vi "Benchmark DMA.vi"() -> ()   [LabVIEW 2016]
uses:
  Controls/Throughput Metrics.ctl
  Controls/Overhead Metrics.ctl
panel:
  in  "Driver":enum16{"Old Driver", "New Driver"}(ring)=enum."New Driver"
  in  "Tab Control":T1(tab)
  out "Channel Counts":i32[](array[numeric])=[1, 10, 100, 1000, 10000, 100000]
  out "Block Write":T2[](array[typedef]) {"Transfer Rate" format="%.2pB/s"; "Duration Std. Dev." format="%.0f µs"; "Duration Average" format="%.0f µs"}
  out "Block Read":T2[](array[typedef]) {"Transfer Rate" format="%.2pB/s"; "Duration Std. Dev." format="%.0f µs"; "Duration Average" format="%.0f µs"}
  out "Scatter-Gather Write":T2[](array[typedef]) {"Transfer Rate" format="%.2pB/s"; "Duration Std. Dev." format="%.0f µs"; "Duration Average" format="%.0f µs"}
  out "Scatter-Gather Read":T2[](array[typedef]) {"Transfer Rate" format="%.2pB/s"; "Duration Std. Dev." format="%.0f µs"; "Duration Average" format="%.0f µs"}
  in  "Tab Control Histograms":enum32{"Block Write", "Page 2"}(tab)
  out "Block Write 100000":T3(graph)
  out "Block Write 10000":T3(graph)
  out "Block Write 1000":T3(graph)
  out "Block Write 100":T3(graph)
  out "Block Write 10":T3(graph)
  out "Block Write 1":T3(graph)
  out "Write Overhead":T4 {"Duration Scatter-Gather" format="%.0f µs"; "Duration N Blocks" format="%.0f µs"; "Duration 1 Block" format="%.0f µs"}
  out "Read Overhead":T4 {"Duration Scatter-Gather" format="%.0f µs"; "Duration N Blocks" format="%.0f µs"; "Duration 1 Block" format="%.0f µs"}
  in  "Channel Count":i32=100000
  in  "Number of Blocks":i32=100
  in  "VISA resource name":refnum<visa-resource-name>
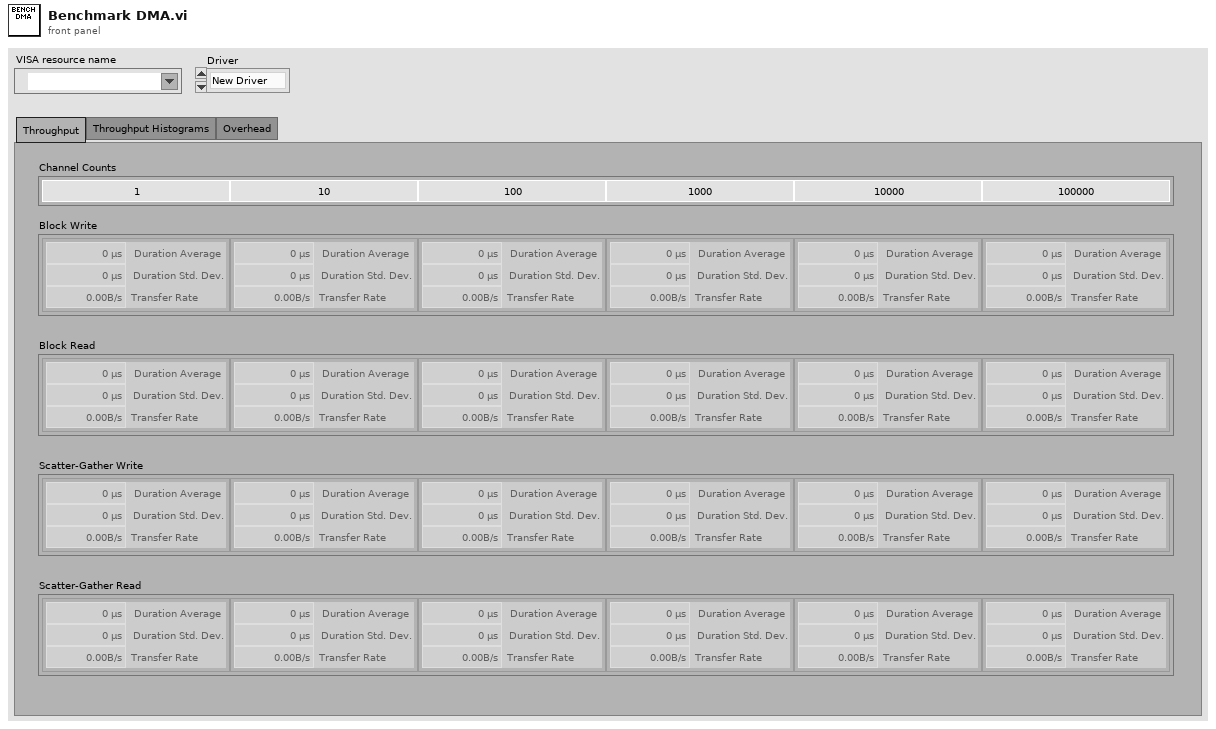
[diagram p1: front panel]
types:
  T1 = enum32{"Throughput", "Throughput Histograms", "Overhead"}
  T2 = typedef "Throughput Metrics.ctl" = cluster{"Duration Average":u32, "Duration Std. Dev.":u32, "Transfer Rate":dbl}
  T3 = cluster{"X Values":dbl[], "Histogram: h(x)":i32[]}
  T4 = typedef "Overhead Metrics.ctl" = cluster{"Duration 1 Block":u32, "Duration N Blocks":u32, "Duration Scatter-Gather":u32}
  T5 = cluster{"X Values":dbl[], "Histogram: h(x)":i32[]}[]
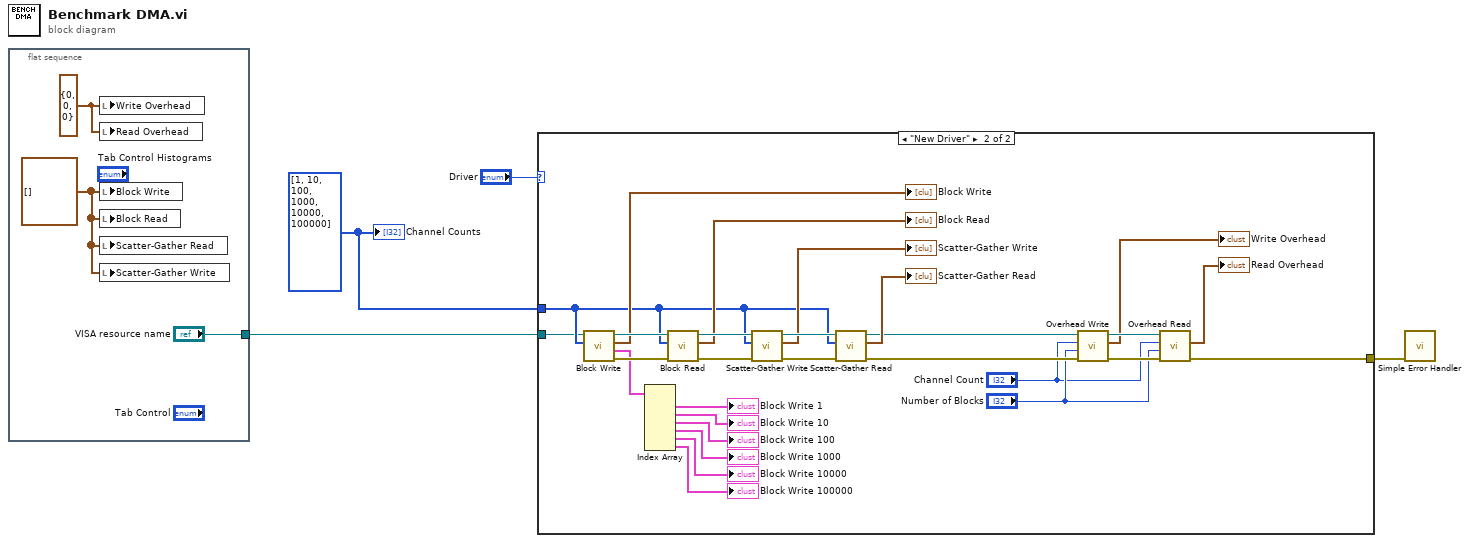
[diagram p0: block diagram]
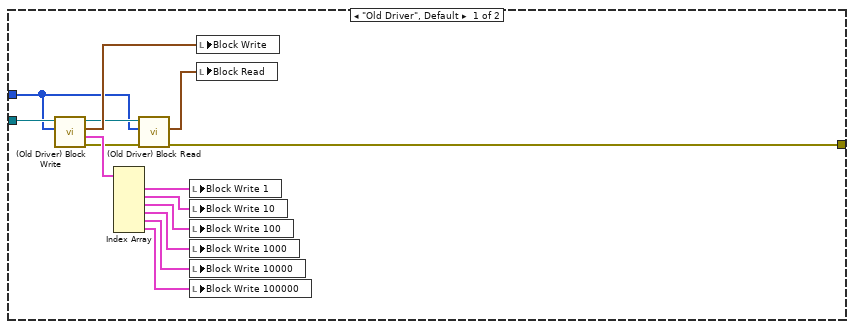
[diagram p2: hidden frame]
diagram:
  w4 = i32[] [1, 10, 100, 1000, 10000, 100000] ("Channel Counts")
  n1 = flat-sequence {
    tunnel: ["VISA resource name"] -> w3
    frame #0 {
      w5 = T4 {"Duration 1 Block"=0, "Duration N Blocks"=0, "Duration Scatter-Gather"=0} ("Write Overhead")
      w7 = T2[] [] ("Block Write")
      n2 = local write "Write Overhead"(w5) -> ()
      n3 = local write "Read Overhead"(w5) -> ()
      n4 = local write "Block Write"(w7) -> ()
      n5 = local write "Block Read"(w7) -> ()
      n6 = local write "Scatter-Gather Read"(w7) -> ()
      n7 = local write "Scatter-Gather Write"(w7) -> ()
    }
  }
  n8 = case shown="\"New Driver\"" "Driver" {
    tunnel: w4 -> [w10 w39]
    tunnel: w3 -> [w21 w30]
    tunnel: [w8 w22] -> w2
    frame "Old Driver", Default {
      n9 = call "(Old Driver) Block Write.vi"("Channel Counts"=w10, "VISA resource name"=w21) -> ("error out"=w11:errorcluster, "Histograms"=w19:T5, "Metrics"=w20:T2[], "VISA resource name out"=w12:refnum<visa-resource-name>)  [unwired: 6 in]
      n10 = Index Array(array=w19) -> (element #1=w18:T3, element #2=w17:T3, element #3=w16:T3, element #4=w15:T3, element #5=w14:T3, element #6=w13:T3)  [unwired: 6 in]
      n11 = call "(Old Driver) Block Read.vi"("error in (no error)"=w11, "Channel Counts"=w10, "VISA resource name"=w12) -> ("error out"=w8:errorcluster, "Metrics"=w9:T2[])  [unwired: 5 in, 2 out]
      n12 = local write "Block Write 1"(w18) -> ()
      n13 = local write "Block Write 10"(w17) -> ()
      n14 = local write "Block Write 100"(w16) -> ()
      n15 = local write "Block Write 1000"(w15) -> ()
      n16 = local write "Block Write 10000"(w14) -> ()
      n17 = local write "Block Write 100000"(w13) -> ()
      n18 = local write "Block Write"(w20) -> ()
      n19 = local write "Block Read"(w9) -> ()
    }
    frame "New Driver" {
      n20 = call "Block Write.vi"("Channel Counts"=w39, "VISA resource name"=w30) -> ("error out"=w48:errorcluster, "Histograms"=w29:T5, "Metrics"=→"Block Write":T2[], "VISA resource name out"=w49:refnum<visa-resource-name>)  [unwired: 6 in]
      n21 = Index Array(array=w29) -> (element #1=→"Block Write 1":T3, element #2=→"Block Write 10":T3, element #3=→"Block Write 100":T3, element #4=→"Block Write 1000":T3, element #5=→"Block Write 10000":T3, element #6=→"Block Write 100000":T3)  [unwired: 6 in]
      n22 = call "Block Read.vi"("error in (no error)"=w48, "Channel Counts"=w39, "VISA resource name"=w49) -> ("error out"=w46:errorcluster, "Metrics"=→"Block Read":T2[], "VISA resource name out"=w47:refnum<visa-resource-name>)  [unwired: 5 in, 1 out]
      n23 = call "Scatter-Gather Write.vi"("error in (no error)"=w46, "Channel Counts"=w39, "VISA resource name"=w47) -> ("error out"=w44:errorcluster, "Metrics"=→"Scatter-Gather Write":T2[], "VISA resource name out"=w45:refnum<visa-resource-name>)  [unwired: 5 in, 1 out]
      n24 = call "Scatter-Gather Read.vi"("error in (no error)"=w44, "Channel Counts"=w39, "VISA resource name"=w45) -> ("error out"=w37:errorcluster, "Metrics"=→"Scatter-Gather Read":T2[], "VISA resource name out"=w38:refnum<visa-resource-name>)  [unwired: 5 in, 1 out]
      n25 = call "Overhead Write.vi"("error in (no error)"=w37, "Number of Blocks"="Number of Blocks", "Channel Count"="Channel Count", "VISA resource name"=w38) -> ("error out"=w35:errorcluster, "Overhead Metrics"=→"Write Overhead":T4, "VISA resource name out"=w36:refnum<visa-resource-name>)  [unwired: 5 in]
      n26 = call "Overhead Read.vi"("error in (no error)"=w35, "Number of Blocks"="Number of Blocks", "Channel Count"="Channel Count", "VISA resource name"=w36) -> ("error out"=w22:errorcluster, "Overhead Metrics"=→"Read Overhead":T4)  [unwired: 5 in, 1 out]
    }
  }
  n27 = call <vilib>:"Simple Error Handler.vi"("error in (no error)"=w2) -> ()  [unwired: 4 in, 5 out]
  "Channel Counts" <- w4
